vi "Averaging for 3.0.vi"(0 "Shorter Name":string, 1 "Timepoints":dbl[](array[numeric]), 2 "Folder to Save":path, 3 "number of y":dbl, 4 "number of x":dbl, 5 "Name of File":string, 6 "Folder Name":string) -> ()   [LabVIEW 2015]
uses:
  <vilib>/Utility/file.llb/Read Delimited Spreadsheet (DBL).vi
  <vilib>/Utility/file.llb/Write Delimited Spreadsheet (DBL).vi
panel:
  out "Diagnostic indicator":dbl
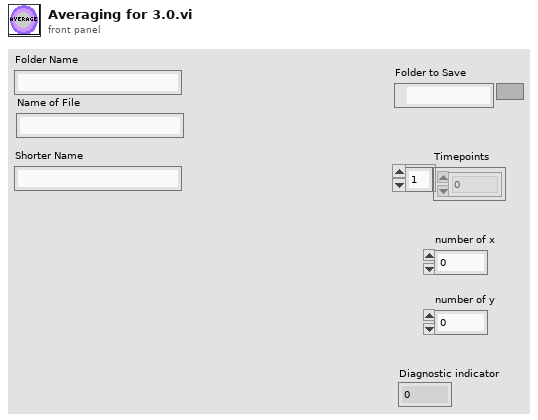
[diagram p1: front panel]
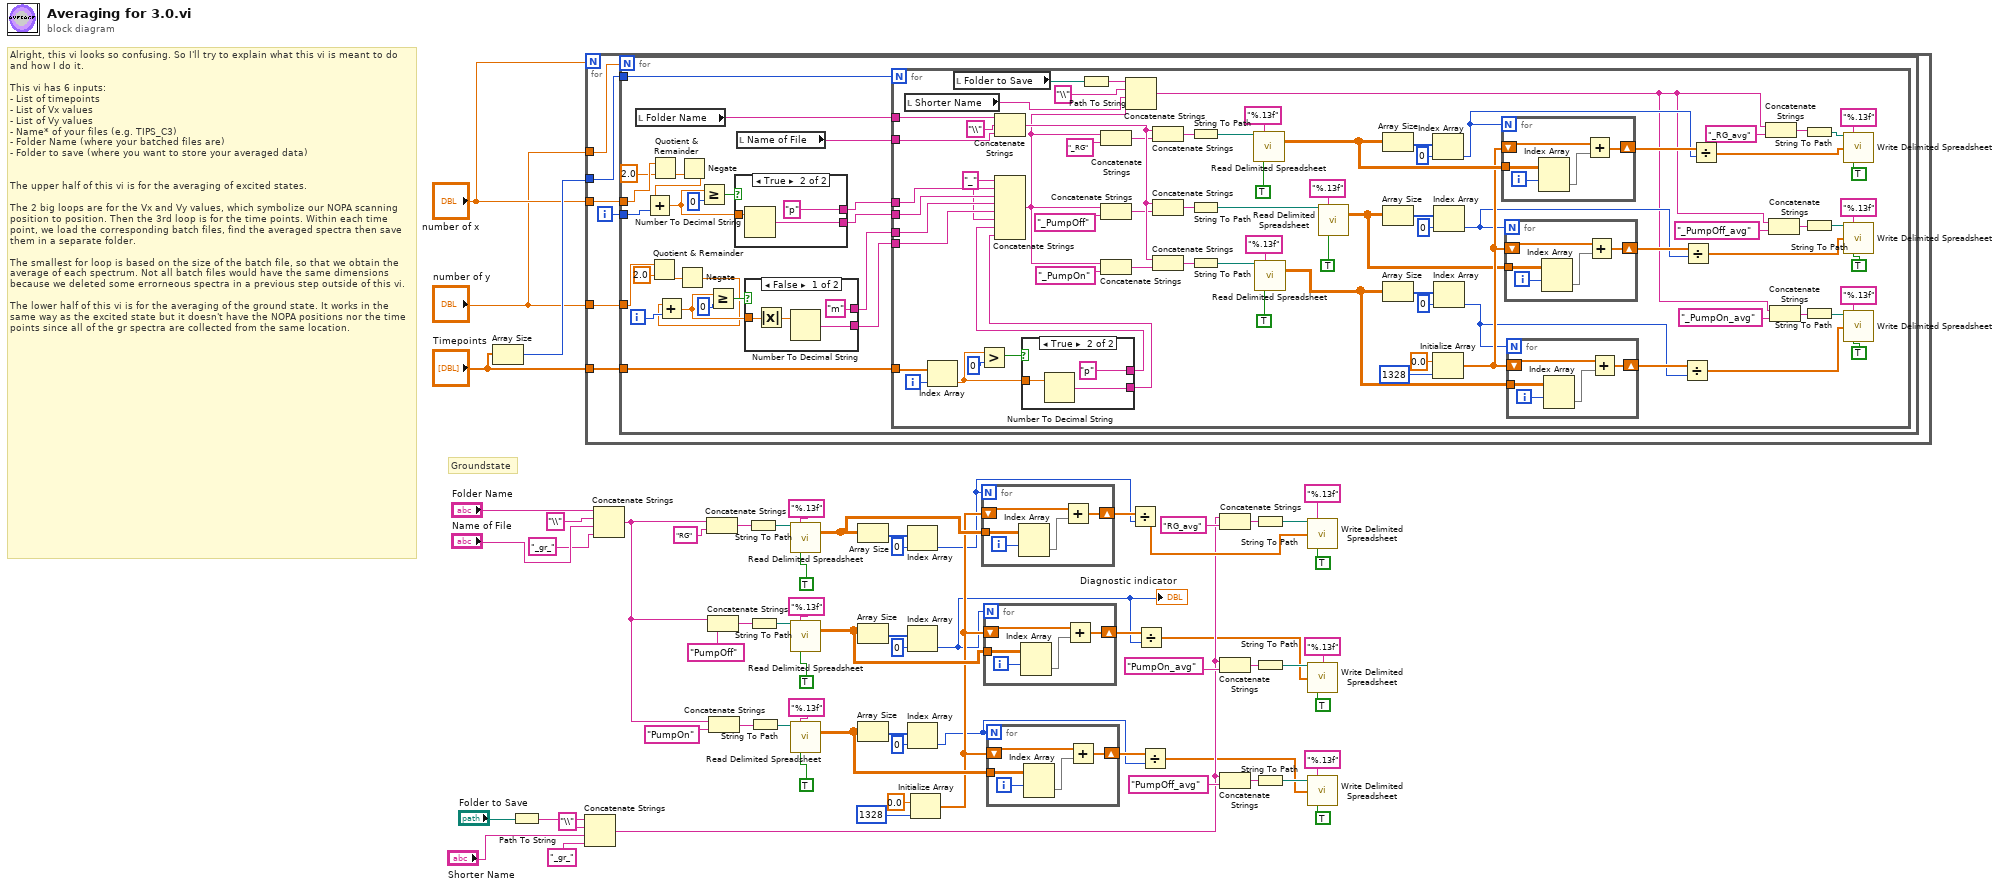
[diagram p0: block diagram]
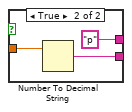
[diagram p2: hidden frame]
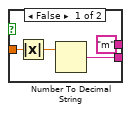
[diagram p3: hidden frame]
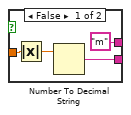
[diagram p4: hidden frame]
diagram:
  # "Groundstate"
  # "Alright, this vi looks so confusing. So I'll try to explain what this vi is meant to do and how I do it.\n\nThis vi has 6 inputs:\n- List of timepoints \n- List of Vx values \n- List of Vy values\n- Name* of your files (e.g. TIPS_C3)\n- Folder Name (where your batched files are)\n- Folder to save (where you want to store your averaged data)\n\n\nThe upper half of this vi is for the averaging of excited states.\n\nThe 2 big loops are for the Vx and Vy values, which symbolize our NOPA scanning position to position. Then the 3rd loop is for the time points. Within each time point, we load the corresponding batch files, find the averaged spectra then save them in a separate folder. \n\nThe smallest for loop is based on the size of the batch file, so that we obtain the average of each spectrum. Not all batch files would have the same dimensions because we deleted some errorneous spectra in a previous step outside of this vi.\n\nThe lower half of this vi is for the averaging of the ground state. It works in the same way as the excited state but it doesn't have the NOPA positions nor the time points since all of the gr spectra are collected from the same location."
  n1 = Array Size(array="Timepoints") -> (size(s)=w66:i32)
  n2 = Path To String(path="Folder to Save") -> (string=w42:string)
  n3 = Concatenate Strings(w42, "\\" ("string"), "Shorter Name", "_gr_" ("string")) -> (w5:string)
  n4 = for {
    N: "number of x" -> [_]
    tunnel: "number of y" -> [w67]
    tunnel: w66 -> [w72]
    tunnel: "number of x" -> [w71]
    tunnel: "number of y" -> [w69]
    tunnel: "Timepoints" -> [w68]
    i -> [w70]
    n5 = for {
      N: w67 -> [_]
      tunnel: w72 -> [w96]
      tunnel: w71 -> [w80]
      tunnel: w70 -> [w93]
      tunnel: w69 -> [w76]
      tunnel: w68 -> [w84]
      i -> [w89]
      n6 = local read "Folder Name"() -> (w82:string)
      n7 = Quotient & Remainder(x=w76, y=2.0) -> (floor(x/y)=w74:dbl)  [unwired: 1 out]
      n8 = Quotient & Remainder(x=w80, y=2.0) -> (floor(x/y)=w78:dbl)  [unwired: 1 out]
      n9 = Negate(x=w74) -> (-x=w73:dbl)
      n10 = Add(x=w73, y=w89) -> (x+y=w90:dbl)
      n11 = Negate(x=w78) -> (-x=w77:dbl)
      n12 = Add(x=w77, y=w93) -> (x+y=w83:dbl)
      n13 = Greater Or Equal?(x=w83, y=0) -> (x >= y?=w94:bool)
      n14 = Greater Or Equal?(x=w90, y=0) -> (x >= y?=w92:bool)
      n15 = case shown="True" w94 {
        tunnel: ["m" "p"] -> w88
        tunnel: w83 -> [w107 w108]
        tunnel: [w105 w109] -> w87
        frame False {
          n16 = Absolute Value(x=w107) -> (abs(x)=w106:dbl)
          n17 = Number To Decimal String(number=w106) -> (decimal integer string=w105:string)  [unwired: 1 in]
        }
        frame True {
          n18 = Number To Decimal String(number=w108) -> (decimal integer string=w109:string)  [unwired: 1 in]
        }
      }
      n19 = local read "Name of File"() -> (w81:string)
      n20 = case shown="False" w92 {
        tunnel: ["m" "p"] -> w86
        tunnel: w90 -> [w99 w101]
        tunnel: [w97 w102] -> w85
        frame False {
          n21 = Absolute Value(x=w99) -> (abs(x)=w98:dbl)
          n22 = Number To Decimal String(number=w98) -> (decimal integer string=w97:string)  [unwired: 1 in]
        }
        frame True {
          n23 = Number To Decimal String(number=w101) -> (decimal integer string=w102:string)  [unwired: 1 in]
        }
      }
      n24 = for {
        N: w96 -> [_]
        tunnel: w81 -> [w112]
        tunnel: w82 -> [w186]
        tunnel: w88 -> [w185]
        tunnel: w87 -> [w169]
        tunnel: w86 -> [w184]
        tunnel: w85 -> [w183]
        tunnel: w84 -> [w179]
        i -> [w178]
        w165 = "_"
        n25 = local read "Shorter Name"() -> (w111:string)
        n26 = Index Array(array=w179, index=w178) -> (element=w181:dbl)
        n27 = local read "Folder to Save"() -> (w121:path)
        n28 = Greater?(x=w181, y=0) -> (0:w180:bool)
        n29 = Concatenate Strings(w186, "\\" ("string"), w112) -> (w161:string)
        n30 = case shown="True" w180 {
          tunnel: ["m" "p"] -> w176
          tunnel: w181 -> [w204 w206]
          tunnel: [w202 w207] -> w177
          frame False {
            n31 = Absolute Value(x=w204) -> (abs(x)=w203:dbl)
            n32 = Number To Decimal String(number=w203) -> (decimal integer string=w202:string)  [unwired: 1 in]
          }
          frame True {
            n33 = Number To Decimal String(number=w206) -> (decimal integer string=w207:string)  [unwired: 1 in]
          }
        }
        n34 = Concatenate Strings(w165, w185, w169, w184, w183, w165, w176, w177) -> (w113:string)
        n35 = Path To String(path=w121) -> (string=w120:string)
        n36 = Concatenate Strings(w113, "_RG" ("string")) -> (w159:string)
        n37 = Concatenate Strings(w113, "_PumpOff" ("string")) -> (w155:string)
        n38 = Concatenate Strings(w113, "_PumpOn" ("string")) -> (w156:string)
        n39 = Concatenate Strings(w120, "\\" ("string"), w111, w113) -> (w117:string)
        n40 = Concatenate Strings(w161, w159) -> (w166:string)
        n41 = Concatenate Strings(w161, w155) -> (w163:string)
        n42 = Concatenate Strings(w161, w156) -> (w162:string)
        n43 = String To Path(string=w166) -> (path=w167:path)
        n44 = String To Path(string=w163) -> (path=w150:path)
        n45 = String To Path(string=w162) -> (path=w149:path)
        n46 = call-poly <vilib>:"Read Delimited Spreadsheet.vi"("file path (dialog if empty)"=w167, "format (%.3f)"="%.13f", "transpose? (F)"=TRUE) -> ("all rows"=w137:dbl[][])  [unwired: 7 in, 5 out]
        n47 = call-poly <vilib>:"Read Delimited Spreadsheet.vi"("file path (dialog if empty)"=w149, "format (%.3f)"="%.13f", "transpose? (F)"=TRUE) -> ("all rows"=w132:dbl[][])  [unwired: 7 in, 5 out]
        n48 = call-poly <vilib>:"Read Delimited Spreadsheet.vi"("file path (dialog if empty)"=w150, "format (%.3f)"="%.13f", "transpose? (F)"=TRUE) -> ("all rows"=w131:dbl[][])  [unwired: 7 in, 5 out]
        n49 = Array Size(array=w137) -> (size(s)=w145:i32[])
        n50 = Array Size(array=w131) -> (size(s)=w141:i32[])
        n51 = Array Size(array=w132) -> (size(s)=w140:i32[])
        n52 = Index Array(array=w145, index=0) -> (element=w135:i32)
        n53 = Initialize Array(0.0 ("element"), 1328 ("dimension size")) -> (w133:dbl[])
        n54 = Index Array(array=w141, index=0) -> (element=w128:i32)
        n55 = Index Array(array=w140, index=0) -> (element=w127:i32)
        n56 = for {
          N: w135 -> [_]
          tunnel: w137 -> [w200]
          shift-right: [w197] -> w136
          shift-left: w133 -> [w198]
          i -> [w201]
          n57 = Index Array(array=w200, index (row)=w201) -> (element=w199:dbl[])  [unwired: 1 in]
          n58 = Add(x=w198, y=w199) -> (x+y=w197:dbl[])
        }
        n59 = for {
          N: w128 -> [_]
          tunnel: w131 -> [w195]
          shift-right: [w192] -> w129
          shift-left: w133 -> [w193]
          i -> [w196]
          n60 = Index Array(array=w195, index (row)=w196) -> (element=w194:dbl[])  [unwired: 1 in]
          n61 = Add(x=w193, y=w194) -> (x+y=w192:dbl[])
        }
        n62 = for {
          N: w127 -> [_]
          tunnel: w132 -> [w190]
          shift-right: [w187] -> w130
          shift-left: w133 -> [w188]
          i -> [w191]
          n63 = Index Array(array=w190, index (row)=w191) -> (element=w189:dbl[])  [unwired: 1 in]
          n64 = Add(x=w188, y=w189) -> (x+y=w187:dbl[])
        }
        n65 = Divide(x=w130, y=w127) -> (x/y=w125:dbl[])
        n66 = Divide(x=w129, y=w128) -> (x/y=w126:dbl[])
        n67 = Divide(x=w136, y=w135) -> (x/y=w134:dbl[])
        n68 = Concatenate Strings(w117, "_RG_avg" ("string")) -> (w124:string)
        n69 = Concatenate Strings(w117, "_PumpOff_avg" ("string")) -> (w119:string)
        n70 = Concatenate Strings(w117, "_PumpOn_avg" ("string")) -> (w118:string)
        n71 = String To Path(string=w124) -> (path=w172:path)
        n72 = String To Path(string=w119) -> (path=w171:path)
        n73 = String To Path(string=w118) -> (path=w170:path)
        n74 = call-poly <vilib>:"Write Delimited Spreadsheet.vi"("file path (dialog if empty)"=w172, "format (%.3f)"="%.13f", "1D data"=w134, "transpose? (F)"=TRUE) -> ()  [unwired: 10 in, 2 out]
        n75 = call-poly <vilib>:"Write Delimited Spreadsheet.vi"("file path (dialog if empty)"=w171, "format (%.3f)"="%.13f", "1D data"=w126, "transpose? (F)"=TRUE) -> ()  [unwired: 10 in, 2 out]
        n76 = call-poly <vilib>:"Write Delimited Spreadsheet.vi"("file path (dialog if empty)"=w170, "format (%.3f)"="%.13f", "1D data"=w125, "transpose? (F)"=TRUE) -> ()  [unwired: 10 in, 2 out]
      }
    }
  }
  n77 = Concatenate Strings("Folder Name", "\\" ("string"), "Name of File", "_gr_") -> (w25:string)
  n78 = Concatenate Strings(w25, "RG" ("string")) -> (w33:string)
  n79 = Concatenate Strings(w25, "PumpOff" ("string")) -> (w39:string)
  n80 = Concatenate Strings(w25, "PumpOn" ("string")) -> (w29:string)
  n81 = String To Path(string=w33) -> (path=w31:path)
  n82 = String To Path(string=w39) -> (path=w37:path)
  n83 = String To Path(string=w29) -> (path=w27:path)
  n84 = call-poly <vilib>:"Read Delimited Spreadsheet.vi"("file path (dialog if empty)"=w31, "format (%.3f)"="%.13f", "transpose? (F)"=TRUE) -> ("all rows"=w15:dbl[][])  [unwired: 7 in, 5 out]
  n85 = call-poly <vilib>:"Read Delimited Spreadsheet.vi"("file path (dialog if empty)"=w37, "format (%.3f)"="%.13f", "transpose? (F)"=TRUE) -> ("all rows"=w14:dbl[][])  [unwired: 7 in, 5 out]
  n86 = call-poly <vilib>:"Read Delimited Spreadsheet.vi"("file path (dialog if empty)"=w27, "format (%.3f)"="%.13f", "transpose? (F)"=TRUE) -> ("all rows"=w13:dbl[][])  [unwired: 7 in, 5 out]
  n87 = Array Size(array=w15) -> (size(s)=w19:i32[])
  n88 = Array Size(array=w14) -> (size(s)=w21:i32[])
  n89 = Array Size(array=w13) -> (size(s)=w17:i32[])
  n90 = Index Array(array=w19, index=0) -> (element=w10:i32)
  n91 = Index Array(array=w21, index=0) -> (element=w2:i32)
  "Diagnostic indicator" <- w2
  n92 = Index Array(array=w17, index=0) -> (element=w7:i32)
  n93 = Initialize Array(0.0 ("element"), 1328 ("dimension size")) -> (w12:dbl[])
  n94 = for {
    N: w10 -> [_]
    tunnel: w15 -> [w212]
    shift-right: [w209] -> w11
    shift-left: w12 -> [w210]
    i -> [w213]
    n95 = Index Array(array=w212, index (row)=w213) -> (element=w211:dbl[])  [unwired: 1 in]
    n96 = Add(x=w210, y=w211) -> (x+y=w209:dbl[])
  }
  n97 = for {
    N: w2 -> [_]
    tunnel: w14 -> [w217]
    shift-right: [w214] -> w9
    shift-left: w12 -> [w215]
    i -> [w218]
    n98 = Index Array(array=w217, index (row)=w218) -> (element=w216:dbl[])  [unwired: 1 in]
    n99 = Add(x=w215, y=w216) -> (x+y=w214:dbl[])
  }
  n100 = for {
    N: w7 -> [_]
    tunnel: w13 -> [w222]
    shift-right: [w219] -> w8
    shift-left: w12 -> [w220]
    i -> [w223]
    n101 = Index Array(array=w222, index (row)=w223) -> (element=w221:dbl[])  [unwired: 1 in]
    n102 = Add(x=w220, y=w221) -> (x+y=w219:dbl[])
  }
  n103 = Divide(x=w11, y=w10) -> (x/y=w6:dbl[])
  n104 = Divide(x=w9, y=w2) -> (x/y=w4:dbl[])
  n105 = Divide(x=w8, y=w7) -> (x/y=w3:dbl[])
  n106 = Concatenate Strings(w5, "RG_avg") -> (w48:string)
  n107 = Concatenate Strings(w5, "PumpOn_avg") -> (w49:string)
  n108 = Concatenate Strings(w5, "PumpOff_avg") -> (w50:string)
  n109 = String To Path(string=w48) -> (path=w52:path)
  n110 = String To Path(string=w49) -> (path=w54:path)
  n111 = String To Path(string=w50) -> (path=w56:path)
  n112 = call-poly <vilib>:"Write Delimited Spreadsheet.vi"("file path (dialog if empty)"=w52, "format (%.3f)"="%.13f", "1D data"=w6, "transpose? (F)"=TRUE) -> ()  [unwired: 10 in, 2 out]
  n113 = call-poly <vilib>:"Write Delimited Spreadsheet.vi"("file path (dialog if empty)"=w54, "format (%.3f)"="%.13f", "1D data"=w4, "transpose? (F)"=TRUE) -> ()  [unwired: 10 in, 2 out]
  n114 = call-poly <vilib>:"Write Delimited Spreadsheet.vi"("file path (dialog if empty)"=w56, "format (%.3f)"="%.13f", "1D data"=w3, "transpose? (F)"=TRUE) -> ()  [unwired: 10 in, 2 out]
